vi "OpenPort.vi"(9 "Baud Rate Input":T2(ring)=enum."115200" caption="Baud Rate", 10 "Port Id Input":T1(ring) caption="Port Name", 11 "Error Input":errorcluster) -> (0 "Uart Output":cluster{u64} {"?" format="%x"}, 1 "Information":string, 2 "Port Status":bool, 3 "Error Output":errorcluster)   [LabVIEW 2019]
doc: "<B>Open</B> a serial port with the given <B>Port Name</B> and <B>Baud Rate</B>. If the port cannot be opened, the <B>Port Status</B> will be set to <B>false</B>."
uses:
  dll/LabViewUart.dll
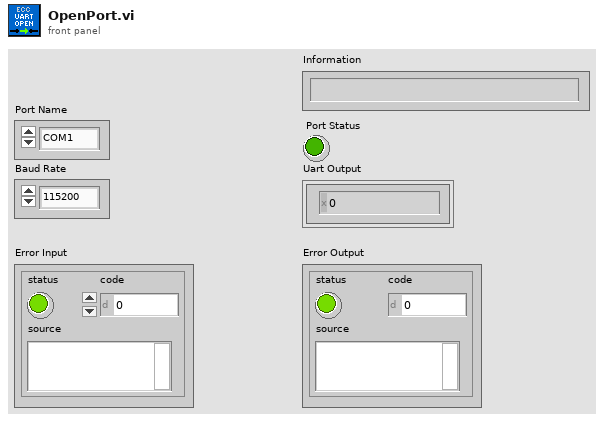
[diagram p1: front panel]
types:
  T1 = enum8{"COM1", "COM2", "COM3", "COM4", "COM5", "COM6", "COM7", "COM8", "COM9", "COM10", "COM11", "COM12", "COM13", "COM14", "COM15", "COM16", "COM17", "COM18", "COM19", "COM20", "COM21", "COM22", "COM23", "COM24", "COM25", "COM26", "COM27", "COM28", "COM29", "COM30", "COM31", "COM32", "COM33", "COM34", "COM35", "COM36", "COM37", "COM38", "COM39", "COM40", "COM41", "COM42", "COM43", "COM44", "COM45", "COM46", "COM47", "COM48"}
  T2 = enum32{"300", "600", "1200", "2400", "4800", "9600", "14400", "19200", "28800", "38400", "56000", "57600", "115200", "128000", "256000"}
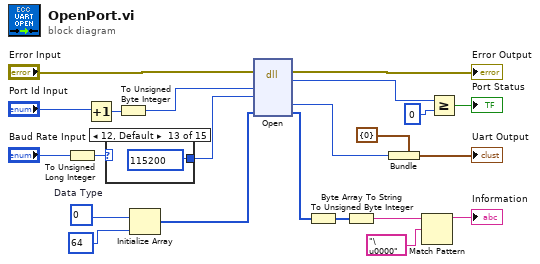
[diagram p0: block diagram]
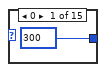
[diagram p2: hidden frame]
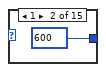
[diagram p3: hidden frame]
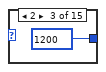
[diagram p4: hidden frame]
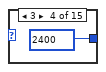
[diagram p5: hidden frame]
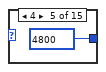
[diagram p6: hidden frame]
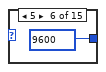
[diagram p7: hidden frame]
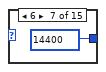
[diagram p8: hidden frame]
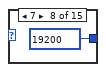
[diagram p9: hidden frame]
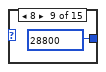
[diagram p10: hidden frame]
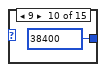
[diagram p11: hidden frame]
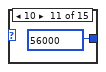
[diagram p12: hidden frame]
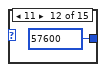
[diagram p13: hidden frame]
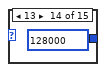
[diagram p14: hidden frame]
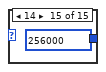
[diagram p15: hidden frame]
diagram:
  w7 = i8 0  # Data Type
  n1 = To Unsigned Long Integer(number="Baud Rate Input") -> (unsigned 32bit integer=w13:u32)
  n2 = Increment(x="Port Id Input") -> (x+1=w15:T1)
  n3 = case shown="12, Default" w13 {
    tunnel: [u32 300 u32 600 u32 1200 u32 2400 u32 4800 u32 9600 u32 14400 u32 19200 u32 28800 u32 38400 u32 56000 u32 57600 u32 115200 u32 128000 u32 256000] -> w12
    frame 0 {
    }
    frame 1 {
    }
    frame 2 {
    }
    frame 3 {
    }
    frame 4 {
    }
    frame 5 {
    }
    frame 6 {
    }
    frame 7 {
    }
    frame 8 {
    }
    frame 9 {
    }
    frame 10 {
    }
    frame 11 {
    }
    frame 12, Default {
    }
    frame 13 {
    }
    frame 14 {
    }
  }
  n4 = To Unsigned Byte Integer(number=w15) -> (unsigned 8bit integer=w17:u8)
  n5 = Initialize Array(w7, 64 ("dimension size")) -> (w8:i8[])
  n6 = dll-call lib="D:/Google Drive/INC-2020/INC352/INC352-2020/LabVIEW/examples/uart-cmdex/SubVI/dll/LabViewUart.dll" fn="Open"(error in="Error Input", "Port Id"=w17, "Baud Rate"=w12, "info"=w8) -> (error out=→"Error Output":errorcluster, "Error Code"=w20:i32, "Uart Handle"=w9:u64, "info"=w5:i8[])  [unwired: 5 in, 1 out]
  n7 = To Unsigned Byte Integer(number=w5) -> (unsigned 8bit integer=w4:u8[])
  n8 = Byte Array To String(unsigned byte array=w4) -> (string=w2:string)
  n9 = Bundle(cluster=cluster{u64} {0}, w9) -> (→"Uart Output":cluster{u64})
  n10 = Match Pattern(string=w2, regular expression="\u0000") -> (before substring=→"Information":string)  [unwired: 1 in, 3 out]
  n11 = Greater Or Equal?(x=w20, y=0) -> (x >= y?=→"Port Status":bool)
